vi "EvaluateConditions.vi"(8 "error in (no error)":errorcluster, 10 "conditions in":T1[](array[typedef])=[{"Condition"={"Source"="", "Type"="", "Operator"="", "CompareTo"="", "DwellSeconds"=0.0}, "LatchValue"="", "LatchTime"=timestamp(0 s since 1904-01-01)}, {"Condition"={"Source"="", "Type"="", "Operator"="", "CompareTo"="", "DwellSeconds"=0.0}, "LatchValue"="", "LatchTime"=timestamp(0 s since 1904-01-01)}], 11 "map":T3) -> (0 "error out":errorcluster, 1 "valid":bool[](array[boolean]), 2 "conditions out":T1[](array[typedef]), 3 "trigger":bool[](array[boolean]))   [LabVIEW 2017, in "Trigger.lvlib"]
uses:
  <vilib>/addons/InsightCM/Devices/Shared/Common/Trigger/Trigger.lvlib
  <vilib>/addons/InsightCM/Devices/Shared/Common/Trigger/controls/TriggerCondition.ctl
  <vilib>/addons/InsightCM/MessageBus/Base/controls/Condition.ctl
  <vilib>/addons/PointValueMap/controls/PointMap.ctl
  <vilib>/addons/PointValueMap/subVIs/Point_Read_double.vi
  <vilib>/addons/PointValueMap/subVIs/Point_Read_i32.vi
  <vilib>/addons/PointValueMap/PointValueMap.lvlib
  <vilib>/addons/InsightCM/Utilities/CronScheduler/CronScheduler.lvlib
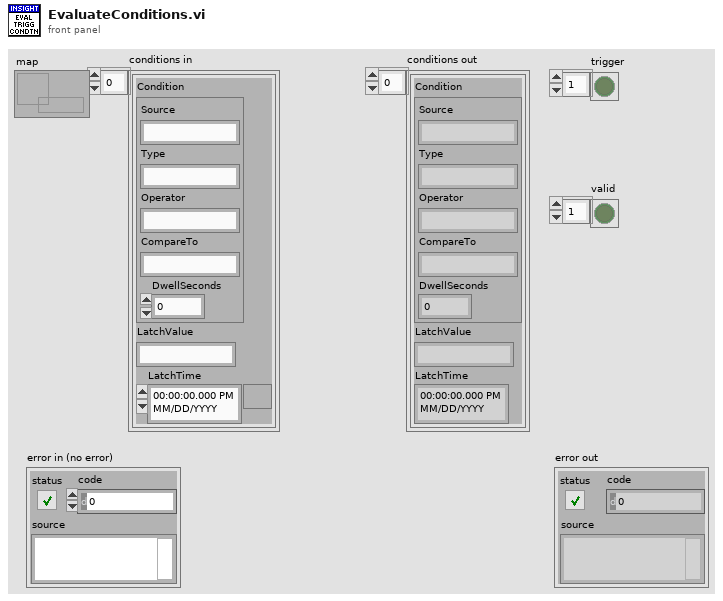
[diagram p1: front panel]
types:
  T1 = typedef "Trigger.lvlib/TriggerCondition.ctl" = cluster{"Condition":T2, "LatchValue":string, "LatchTime":timestamp}
  T2 = typedef "Condition.ctl" = cluster{"Source":string, "Type":string, "Operator":string, "CompareTo":string, "DwellSeconds":dbl}
  T3 = typedef "PointValueMap.lvlib/PointMap.ctl" = refnum<data-value>
  T4 = typedef "CronScheduler.lvlib/CronSchedule.ctl" = cluster{"minutes":string, "hours":string, "day of month":string, "month":string, "day of week":string, "year":string}
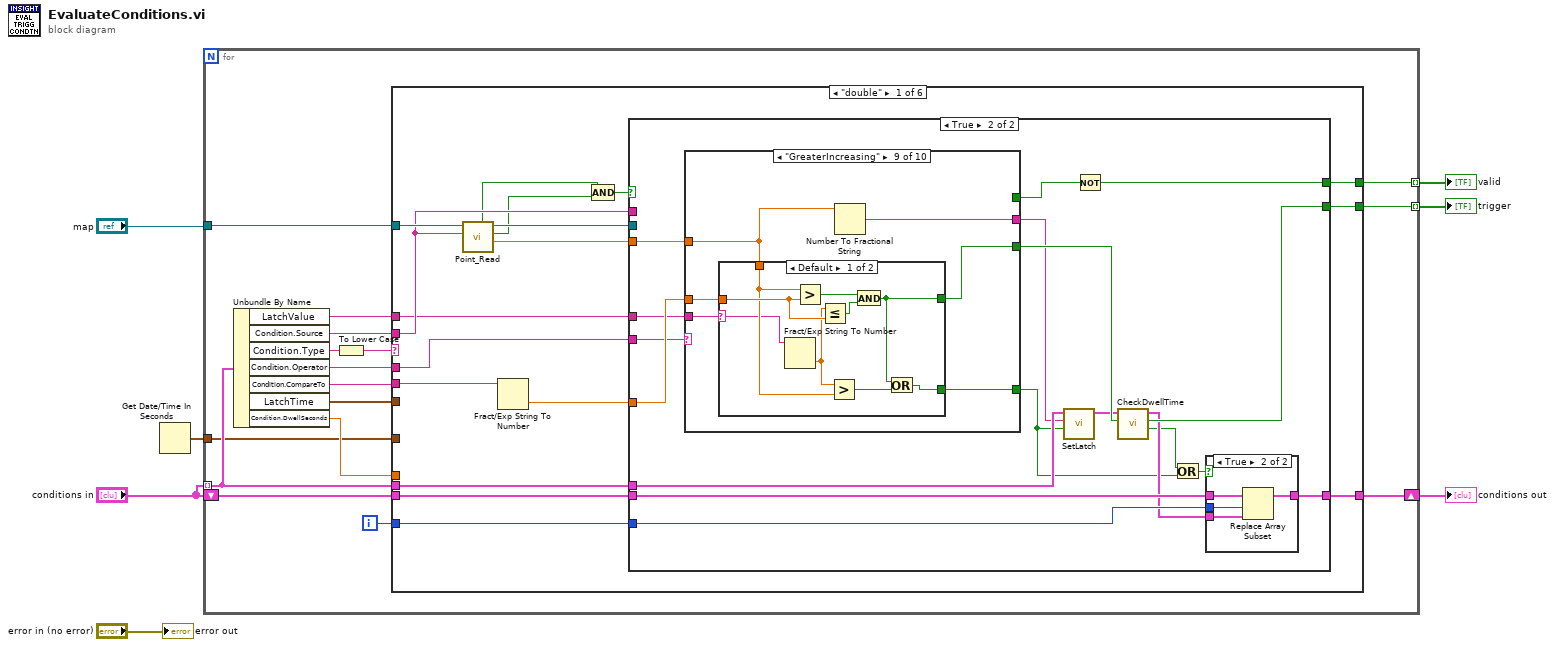
[diagram p0: block diagram]
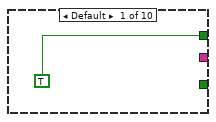
[diagram p4: hidden frame]
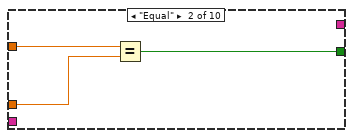
[diagram p5: hidden frame]
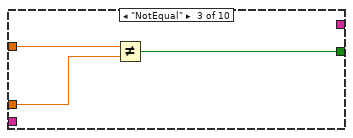
[diagram p6: hidden frame]
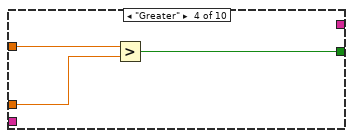
[diagram p7: hidden frame]
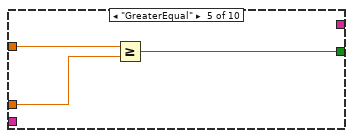
[diagram p8: hidden frame]
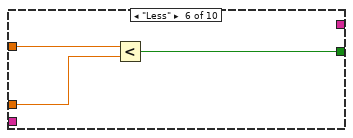
[diagram p9: hidden frame]
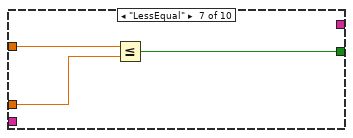
[diagram p10: hidden frame]
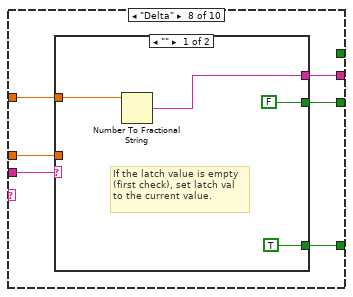
[diagram p11: hidden frame]
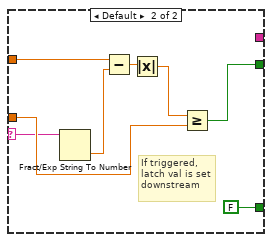
[diagram p12: hidden frame]
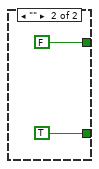
[diagram p13: hidden frame]
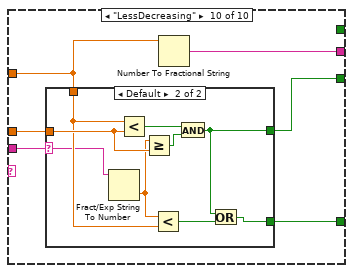
[diagram p14: hidden frame]
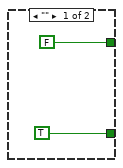
[diagram p15: hidden frame]
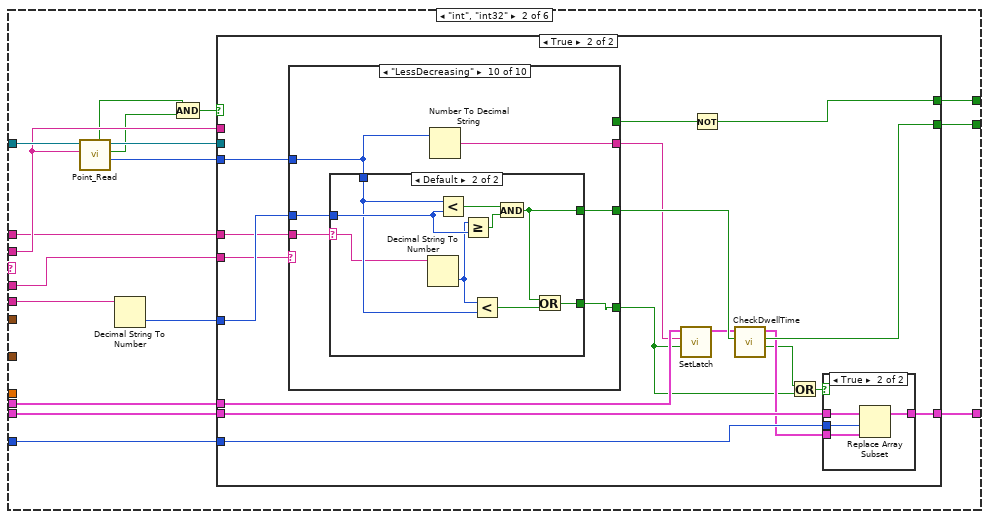
[diagram p16: hidden frame]
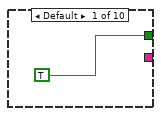
[diagram p19: hidden frame]
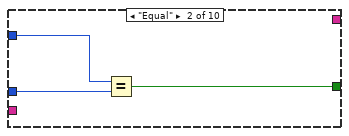
[diagram p20: hidden frame]
diagram:
  n1 = Get Date/Time In Seconds() -> (seconds since 1Jan1904=w2:timestamp)
  n2 = for {
    tunnel: "conditions in" -> [w15] mode=indexing
    tunnel: "map" -> [w19]
    tunnel: [w17] -> w6 mode=indexing
    shift-right: [w12] -> w5
    shift-left: "conditions in" -> [w13]
    tunnel: [w10] -> w4 mode=indexing
    tunnel: w2 -> [w8]
    i -> [w14]
    n3 = Unbundle By Name(w15) -> ("LatchValue"=w16:string, "Condition.Source"=w18:string, "Condition.Type"=w23:string, "Condition.Operator"=w22:string, "Condition.CompareTo"=w21:string, "LatchTime"=w9:timestamp, "Condition.DwellSeconds"=w11:dbl)
    n4 = To Lower Case(string=w23) -> (all lower case string=w20:string)
    n5 = case shown="\"double\"" w20 {
      tunnel: w22 -> [w39 w151 _ w278 _ _]
      tunnel: w21 -> [w25 w137 w259 w276 w304 _]
      tunnel: [w38 w150 w250 w277 w305 _] -> w17
      tunnel: w19 -> [w40 w152 _ w275 w300 _]
      tunnel: w18 -> [w37 w149 _ w274 w302 _]
      tunnel: w16 -> [w35 w147 _ _ _ _]
      tunnel: w15 -> [w34 w146 w253 _ _ _]
      tunnel: w14 -> [w33 w145 w254 _ _ _]
      tunnel: w13 -> [w32 w144 w256 w273 w303 w306]
      tunnel: [w31 w143 w255 w273 w303 w306] -> w12
      tunnel: w11 -> [_ _ _ _ _ _]
      tunnel: [w26 w138 TRUE w269 w292 _] -> w10
      tunnel: w9 -> [_ _ w252 _ _ _]
      tunnel: w8 -> [_ _ w249 _ _ _]
      frame "double" {
        n6 = call-poly <vilib>:"Point_Read.vi"("Tag"=w37, "Map"=w40) -> ("Value"=w30:dbl, "Found?"=w29:bool, "Map Out"=w36:T3, "Valid?"=w28:bool)  [unwired: 4 in, 2 out]
        n7 = Fract/Exp String To Number(string=w25) -> (number=w24:dbl)  [unwired: 3 in, 1 out]
        n8 = Compound Arithmetic op=AND(w28, w29) -> (w27:bool)
        n9 = case shown="True" w27 {
          tunnel: w39 -> [_ w52]
          tunnel: [_ w53] -> w38
          tunnel: w37 -> [_ _]
          tunnel: w24 -> [_ w58]
          tunnel: w36 -> [_ _]
          tunnel: w35 -> [_ w51]
          tunnel: w34 -> [_ w47]
          tunnel: w33 -> [_ w55]
          tunnel: w32 -> [w41 w56]
          tunnel: [w41 w54] -> w31
          tunnel: w30 -> [_ w59]
          tunnel: [_ w49] -> w26
          frame False {
            # "Source or compare to tag not valid or found in PVM"
          }
          frame True {
            n10 = case shown="\"GreaterIncreasing\"" w52 {
              tunnel: w59 -> [_ w68 w71 w74 w77 w80 w83 w88 w106 w123]
              tunnel: w58 -> [_ w67 w70 w73 w76 w79 w82 w87 w107 w124]
              tunnel: [_ w66 w69 w72 w75 w78 w81 w89 w104 w121] -> w57
              tunnel: w51 -> [_ _ _ _ _ _ _ w86 w103 w120]
              tunnel: [_ _ _ _ _ _ _ w84 w105 w122] -> w43
              tunnel: [TRUE _ _ _ _ _ _ _ _ _] -> w50
              tunnel: [_ _ _ _ _ _ _ w85 w102 w119] -> w42
              frame Default {
              }
              frame "Equal" {
                n11 = Equal?(x=w68, y=w67) -> (x = y?=w66:bool)
              }
              frame "NotEqual" {
                n12 = Not Equal?(x=w71, y=w70) -> (x != y?=w69:bool)
              }
              frame "Greater" {
                n13 = Greater?(x=w74, y=w73) -> (0:w72:bool)
              }
              frame "GreaterEqual" {
                n14 = Greater Or Equal?(x=w77, y=w76) -> (x >= y?=w75:bool)
              }
              frame "Less" {
                n15 = Less?(x=w80, y=w79) -> (x < y?=w78:bool)
              }
              frame "LessEqual" {
                n16 = Less Or Equal?(x=w83, y=w82) -> (x <= y?=w81:bool)
              }
              frame "Delta" {
                n17 = case shown="\"\"" w86 {
                  selector: w86 -> [_ w95]
                  tunnel: [FALSE w99] -> w89
                  tunnel: w88 -> [w91 w98]
                  tunnel: w87 -> [_ w96]
                  tunnel: [TRUE FALSE] -> w85
                  tunnel: [w90 _] -> w84
                  frame "" {
                    # "If the latch value is empty\n(first check), set latch val\nto the current value."
                    n18 = Number To Fractional String(number=w91) -> (F-format string=w90:string)  [unwired: 3 in]
                  }
                  frame Default {
                    # "If triggered,\nlatch val is set\ndownstream"
                    n19 = Fract/Exp String To Number(string=w95) -> (number=w97:dbl)  [unwired: 3 in, 1 out]
                    n20 = Subtract(x=w98, y=w97) -> (x-y=w101:dbl)
                    n21 = Absolute Value(x=w101) -> (abs(x)=w100:dbl)
                    n22 = Greater Or Equal?(x=w100, y=w96) -> (x >= y?=w99:bool)
                  }
                }
              }
              frame "GreaterIncreasing" {
                n23 = case shown="Default" w103 {
                  selector: w103 -> [w111 _]
                  tunnel: w107 -> [w114 _]
                  tunnel: w106 -> [w113 _]
                  tunnel: [w109 FALSE] -> w104
                  tunnel: [w108 TRUE] -> w102
                  frame Default {
                    n24 = Fract/Exp String To Number(string=w111) -> (number=w112:dbl)  [unwired: 3 in, 1 out]
                    n25 = Greater?(x=w113, y=w114) -> (0:w116:bool)
                    n26 = Less Or Equal?(x=w112, y=w114) -> (x <= y?=w115:bool)
                    n27 = Greater?(x=w112, y=w113) -> (0:w110:bool)
                    n28 = And(x=w116, y=w115) -> (x .and. y?=w109:bool)
                    n29 = Or(x=w109, y=w110) -> (x .or. y?=w108:bool)
                  }
                  frame "" {
                  }
                }
                n30 = Number To Fractional String(number=w106) -> (F-format string=w105:string)  [unwired: 3 in]
              }
              frame "LessDecreasing" {
                n31 = case shown="Default" w120 {
                  selector: w120 -> [_ w130]
                  tunnel: w124 -> [_ w133]
                  tunnel: w123 -> [_ w132]
                  tunnel: [TRUE w127] -> w119
                  tunnel: [FALSE w129] -> w121
                  frame "" {
                  }
                  frame Default {
                    n32 = Fract/Exp String To Number(string=w130) -> (number=w131:dbl)  [unwired: 3 in, 1 out]
                    n33 = Less?(x=w132, y=w133) -> (x < y?=w135:bool)
                    n34 = Greater Or Equal?(x=w131, y=w133) -> (x >= y?=w134:bool)
                    n35 = Less?(x=w131, y=w132) -> (x < y?=w128:bool)
                    n36 = And(x=w135, y=w134) -> (x .and. y?=w129:bool)
                    n37 = Or(x=w129, y=w128) -> (x .or. y?=w127:bool)
                  }
                }
                n38 = Number To Fractional String(number=w123) -> (F-format string=w122:string)  [unwired: 3 in]
              }
            }
            n39 = call <vilib>:"SetLatch.vi"("latch"=w42, "latch value"=w43, "condition in"=w47) -> ("condition out"=w46:T1)  [unwired: 8 in]
            n40 = Not(x=w50) -> (.not. x?=w49:bool)
            n41 = call <vilib>:"CheckDwellTime.vi"("trigger in"=w57, "condition in"=w46) -> ("updated"=w45:bool, "trigger out"=w53:bool, "condition out"=w48:T1)  [unwired: 7 in]
            n42 = Or(x=w45, y=w42) -> (x .or. y?=w44:bool)
            n43 = case shown="True" w44 {
              tunnel: w56 -> [w60 w64]
              tunnel: w55 -> [_ w63]
              tunnel: [w60 w62] -> w54
              tunnel: w48 -> [_ w61]
              frame False {
              }
              frame True {
                n44 = Replace Array Subset(array=w64, new element=w61, index=w63) -> (w62:T1[])
              }
            }
          }
        }
      }
      frame "int", "int32" {
        n45 = call-poly <vilib>:"Point_Read.vi"("Tag"=w149, "Map"=w152) -> ("Value"=w142:i32, "Found?"=w141:bool, "Map Out"=w148:T3, "Valid?"=w140:bool)  [unwired: 4 in, 2 out]
        n46 = Decimal String To Number(string=w137) -> (number=w136:i32)  [unwired: 2 in, 1 out]
        n47 = Compound Arithmetic op=AND(w140, w141) -> (w139:bool)
        n48 = case shown="True" w139 {
          tunnel: w151 -> [_ w164]
          tunnel: [_ w165] -> w150
          tunnel: w149 -> [_ _]
          tunnel: w136 -> [_ w170]
          tunnel: w148 -> [_ _]
          tunnel: w147 -> [_ w163]
          tunnel: w146 -> [_ w159]
          tunnel: w145 -> [_ w167]
          tunnel: w144 -> [w153 w168]
          tunnel: [w153 w166] -> w143
          tunnel: w142 -> [_ w171]
          tunnel: [_ w161] -> w138
          frame False {
            # "Source or compare to tag not valid or found in PVM"
          }
          frame True {
            n49 = case shown="\"LessDecreasing\"" w164 {
              tunnel: w171 -> [_ w180 w183 w186 w189 w192 w195 w200 w218 w235]
              tunnel: w170 -> [_ w179 w182 w185 w188 w191 w194 w199 w219 w236]
              tunnel: [_ w178 w181 w184 w187 w190 w193 w201 w216 w233] -> w169
              tunnel: w163 -> [_ _ _ _ _ _ _ w198 w215 w232]
              tunnel: [_ _ _ _ _ _ _ w196 w217 w234] -> w155
              tunnel: [TRUE _ _ _ _ _ _ _ _ _] -> w162
              tunnel: [_ _ _ _ _ _ _ w197 w214 w231] -> w154
              frame Default {
              }
              frame "Equal" {
                n50 = Equal?(x=w180, y=w179) -> (x = y?=w178:bool)
              }
              frame "NotEqual" {
                n51 = Not Equal?(x=w183, y=w182) -> (x != y?=w181:bool)
              }
              frame "Greater" {
                n52 = Greater?(x=w186, y=w185) -> (0:w184:bool)
              }
              frame "GreaterEqual" {
                n53 = Greater Or Equal?(x=w189, y=w188) -> (x >= y?=w187:bool)
              }
              frame "Less" {
                n54 = Less?(x=w192, y=w191) -> (x < y?=w190:bool)
              }
              frame "LessEqual" {
                n55 = Less Or Equal?(x=w195, y=w194) -> (x <= y?=w193:bool)
              }
              frame "Delta" {
                n56 = case shown="\"False\"" w198 {
                  selector: w198 -> [_ w207]
                  tunnel: [FALSE w211] -> w201
                  tunnel: w200 -> [w205 w210]
                  tunnel: w199 -> [_ w208]
                  tunnel: [TRUE FALSE] -> w197
                  tunnel: [w204 _] -> w196
                  frame "False" {
                    # "If the latch value is empty\n(first check), set latch val\nto the current value."
                    n57 = Number To Decimal String(number=w205) -> (decimal integer string=w204:string)  [unwired: 1 in]
                  }
                  frame Default {
                    # "If triggered,\nlatch val is set\ndownstream"
                    n58 = Decimal String To Number(string=w207) -> (number=w209:i32)  [unwired: 2 in, 1 out]
                    n59 = Subtract(x=w210, y=w209) -> (x-y=w213:i32)
                    n60 = Absolute Value(x=w213) -> (abs(x)=w212:i32)
                    n61 = Greater Or Equal?(x=w212, y=w208) -> (x >= y?=w211:bool)
                  }
                }
              }
              frame "GreaterIncreasing" {
                n62 = case shown="Default" w215 {
                  selector: w215 -> [_ w225]
                  tunnel: w219 -> [_ w228]
                  tunnel: w218 -> [_ w227]
                  tunnel: [TRUE w222] -> w214
                  tunnel: [FALSE w223] -> w216
                  frame "" {
                  }
                  frame Default {
                    n63 = Decimal String To Number(string=w225) -> (number=w226:i32)  [unwired: 2 in, 1 out]
                    n64 = Greater?(x=w227, y=w228) -> (0:w230:bool)
                    n65 = Less Or Equal?(x=w226, y=w228) -> (x <= y?=w229:bool)
                    n66 = Greater?(x=w226, y=w227) -> (0:w224:bool)
                    n67 = And(x=w230, y=w229) -> (x .and. y?=w223:bool)
                    n68 = Or(x=w223, y=w224) -> (x .or. y?=w222:bool)
                  }
                }
                n69 = Number To Decimal String(number=w218) -> (decimal integer string=w217:string)  [unwired: 1 in]
              }
              frame "LessDecreasing" {
                n70 = case shown="Default" w232 {
                  selector: w232 -> [_ w242]
                  tunnel: w236 -> [_ w245]
                  tunnel: w235 -> [_ w244]
                  tunnel: [FALSE w241] -> w233
                  tunnel: [TRUE w239] -> w231
                  frame "" {
                  }
                  frame Default {
                    n71 = Decimal String To Number(string=w242) -> (number=w243:i32)  [unwired: 2 in, 1 out]
                    n72 = Less?(x=w244, y=w245) -> (x < y?=w247:bool)
                    n73 = Greater Or Equal?(x=w243, y=w245) -> (x >= y?=w246:bool)
                    n74 = Less?(x=w243, y=w244) -> (x < y?=w240:bool)
                    n75 = And(x=w247, y=w246) -> (x .and. y?=w241:bool)
                    n76 = Or(x=w241, y=w240) -> (x .or. y?=w239:bool)
                  }
                }
                n77 = Number To Decimal String(number=w235) -> (decimal integer string=w234:string)  [unwired: 1 in]
              }
            }
            n78 = call <vilib>:"SetLatch.vi"("latch"=w154, "latch value"=w155, "condition in"=w159) -> ("condition out"=w158:T1)  [unwired: 8 in]
            n79 = Not(x=w162) -> (.not. x?=w161:bool)
            n80 = call <vilib>:"CheckDwellTime.vi"("trigger in"=w169, "condition in"=w158) -> ("updated"=w157:bool, "trigger out"=w165:bool, "condition out"=w160:T1)  [unwired: 7 in]
            n81 = Or(x=w157, y=w154) -> (x .or. y?=w156:bool)
            n82 = case shown="True" w156 {
              tunnel: w168 -> [w172 w176]
              tunnel: w167 -> [_ w175]
              tunnel: [w172 w174] -> w166
              tunnel: w160 -> [_ w173]
              frame False {
              }
              frame True {
                n83 = Replace Array Subset(array=w176, new element=w173, index=w175) -> (w174:T1[])
              }
            }
          }
        }
      }
      frame "timespanseconds" {
        n84 = Subtract(x=w249, y=w252) -> (x-y=w251:dbl)
        n85 = Decimal String To Number(string=w259, default (0L)=0.0) -> (number=w257:dbl)  [unwired: 1 in, 1 out]
        n86 = Greater?(x=w251, y=w257) -> (0:w250:bool)
        n87 = case shown="True" w250 {
          tunnel: w256 -> [w260 w265]
          tunnel: [w260 w264] -> w255
          tunnel: w254 -> [_ w263]
          tunnel: w253 -> [_ w262]
          tunnel: w249 -> [_ w261]
          frame False {
          }
          frame True {
            n88 = Bundle By Name(cluster=w262, "LatchTime"=w261) -> (w266:T1)
            n89 = Replace Array Subset(array=w265, new element=w266, index=w263) -> (w264:T1[])
          }
        }
      }
      frame "string" {
        n90 = call <vilib>:"Point_Read_string.vi"("Tag"=w274, "Map"=w275) -> ("Error Out"=w267:errorcluster, "Value"=w272:string, "Found?"=w270:bool, "Valid?"=w271:bool)  [unwired: 4 in, 2 out]
        n91 = Compound Arithmetic op=AND(w271, w270, invert w267) -> (w268:bool)
        n92 = case shown="True" w268 {
          tunnel: w278 -> [_ w283]
          tunnel: [_ w282] -> w277
          tunnel: w276 -> [_ w281]
          tunnel: w272 -> [_ w280]
          tunnel: [_ w279] -> w269
          frame False {
          }
          frame True {
            n93 = case shown="\"NotEqual\"" w283 {
              tunnel: w281 -> [w287 w291 _]
              tunnel: [w286 w290 _] -> w282
              tunnel: w280 -> [w285 w289 _]
              tunnel: [TRUE TRUE _] -> w279
              frame "Equal" {
                n94 = Equal?(x=w285, y=w287) -> (x = y?=w286:bool)
              }
              frame "NotEqual" {
                n95 = Not Equal?(x=w289, y=w291) -> (x != y?=w290:bool)
              }
              frame Default {
              }
            }
          }
        }
      }
      frame "cron" {
        # "Subtract offset from incoming\ntimestamp in order to delay\ntrigger by timeTriggerOffset"
        n96 = call-poly <vilib>:"Point_Read.vi"("Tag"="CronOffset", "Map"=w300) -> ("Error Out"=w299:errorcluster, "Value"=w297:dbl)  [unwired: 4 in, 4 out]
        n97 = Get Date/Time In Seconds() -> (seconds since 1Jan1904=w296:timestamp)
        n98 = call <vilib>:"ConvertCronToSchedule.vi"("CRON expression"=w304) -> ("chronSchedule"=w301:T4)  [unwired: 9 in, 1 out]
        n99 = Subtract(x=w296, y=w297) -> (x-y=w295:timestamp)
        n100 = call <vilib>:"CronScheduler.vi"("error in (no error)"=w299, "chron schedule"=w301, "timestamp"=w295, "cron id"=w302) -> ("error out"=w294:errorcluster, "event elapsed"=w305:bool)  [unwired: 6 in]
        n101 = Unbundle By Name(w294) -> ("status"=w293:bool)
        n102 = Not(x=w293) -> (.not. x?=w292:bool)
      }
      frame Default {
      }
    }
  }
  "trigger" <- w6
  "conditions out" <- w5
  "valid" <- w4
  "error out" <- "error in (no error)"
